vi "Accumulate.vi"(6 "reset":bool, 7 "max size":dbl=2147483647.0, 10 "index":i32, 11 "data":dbl[](array[numeric])) -> (3 "data out":dbl[](array[numeric]))   [LabVIEW 2012]
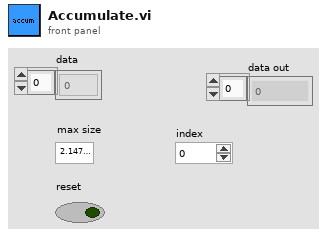
[diagram p1: front panel]
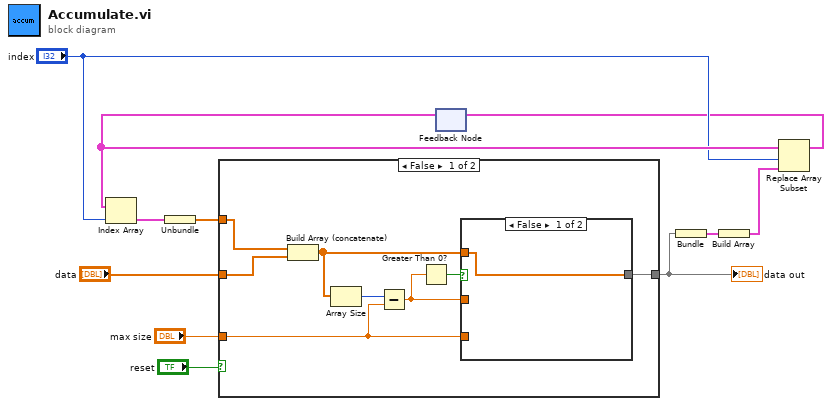
[diagram p0: block diagram]
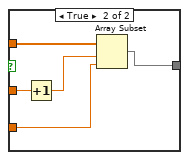
[diagram p2: hidden frame]
diagram:
  n1 = feedback #1() -> (w4:cluster{"data":dbl[]}[])  [unwired: 1 in]
  n2 = Index Array(array=w4, index="index") -> (element=w6:cluster{"data":dbl[]})
  n3 = Unbundle(w6) -> ("data"=w5:dbl[])
  n4 = case shown="False" "reset" {
    tunnel: "data" -> [w18 w25]
    tunnel: [w12 w25] -> w7
    tunnel: "max size" -> [w13 _]
    tunnel: w5 -> [w11 _]
    frame False {
      n5 = Build Array (concatenate)(w11, w18) -> (w17:dbl[])
      n6 = Array Size(array=w17) -> (size(s)=w16:i32)
      n7 = Subtract(x=w16, y=w13) -> (x-y=w14:dbl)
      n8 = Greater Than 0?(x=w14) -> (x > 0?=w15:bool)
      n9 = case shown="False" w15 {
        tunnel: w17 -> [w19 w24]
        tunnel: w14 -> [_ w23]
        tunnel: w13 -> [_ w21]
        tunnel: [w19 w20] -> w12
        frame False {
        }
        frame True {
          n10 = Increment(x=w23) -> (x+1=w22:dbl)
          n11 = Array Subset(array=w24, index=w22, length=w21) -> (w20:dbl[])
        }
      }
    }
    frame True {
    }
  }
  "data out" <- w7
  n12 = Bundle("data"=w7) -> (w2:cluster{"data":dbl[]})  [unwired: 1 in]
  n13 = Build Array(w2) -> ()  [unwired: 1 out]
  n14 = Replace Array Subset(array=w4, new element=w2, index="index") -> (w1:cluster{"data":dbl[]}[])
  n15 = feedback-in #1(w1) -> ()
